vi "LogError.vi"(8 "error in (no error)":errorcluster, 10 "log string":string, 11 "service in":refnum<class "IcmMessageService.lvclass">) -> (0 "error out":errorcluster, 3 "service out":refnum<class "IcmMessageService.lvclass">)   [LabVIEW 2017, in "IcmMessageService.lvclass"]
doc: "Logs a tracepoint instance that includes the error code and the source of an error within an error cluster."
uses:
  <vilib>/addons/InsightCM/MessageBus/MessageService/IcmMessageService.lvclass
  <vilib>/addons/InsightCM/MessageBus/MessageService/IcmMessageService.lvclass/IcmMessageService.ctl
  C:/Program Files (x86)/National Instruments/LabVIEW 2017/vi.lib/addons/InsightCM/Binaries/LabviewMessageAdapter.dll
  Binaries/LabviewMessageAdapter.dll
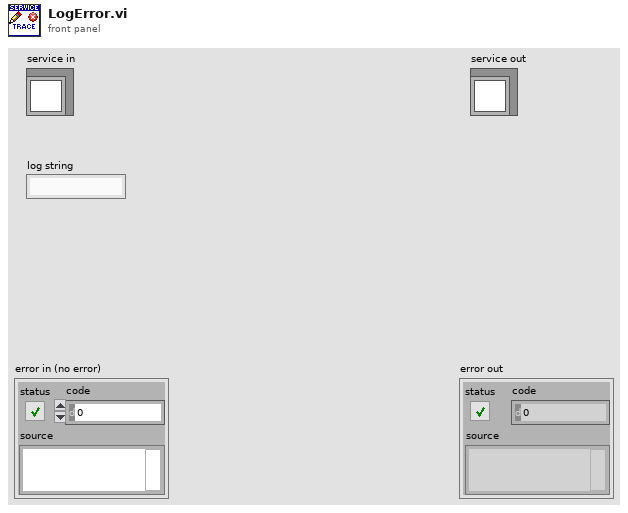
[diagram p1: front panel]
types:
  T1 = typedef "MessageServiceDvr.ctl" = refnum<data-value>
  T2 = typedef "MessageServiceData.ctl" = cluster{"Service":refnum<k24>}
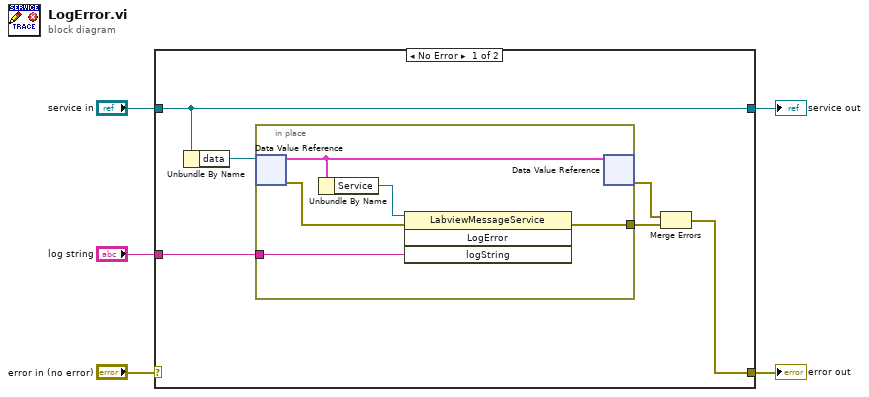
[diagram p0: block diagram]
diagram:
  n1 = case shown="No Error" "error in (no error)" {
    selector: "error in (no error)" -> [_ w18]
    tunnel: [w7 w18] -> w4
    tunnel: [w11 w17] -> w2
    tunnel: "service in" -> [w11 w17]
    tunnel: "log string" -> [w6 _]
    frame No Error {
      n2 = Unbundle By Name(w11) -> ("data"=w10:T1)
      n3 = in-place {
        in-place-border: [w13] -> w8
        in-place-border: w6 -> [w12]
        n4 = in-place-dvr #1(w10) -> (w16:T2, w14:errorcluster)
        n5 = Unbundle By Name(w16) -> ("Service"=w15:refnum<k24>)
        n6 = invoke class="LabviewMessageService" method="LogError"(reference=w15, error in=w14, "logString"=w12) -> (error out=w13:errorcluster)  [unwired: 1 in, 3 out]
        n7 = in-place-dvr #1(w16) -> (w9:errorcluster)  [unwired: 1 out]
      }
      n8 = Merge Errors(w9, w8) -> (w7:errorcluster)
    }
    frame Error {
    }
  }
  "error out" <- w4
  "service out" <- w2
